vi "Enque(waveforms).vi"(7 "at front (F)":bool, 8 "error in":errorcluster, 9 "Message Payload waveforms":waveform(dbl)[](array[waveform]), 10 "Message Command":string, 11 "Message que":T1) -> (0 "error out":errorcluster, 3 "Message que out":T1)   [LabVIEW 2017]
doc: "Transmit a message with a waveform array payload.\nFor a regular message, enqueue the message. For a priority message, enqueue it at the front of the queue.\n\nBolder Software LLC"
uses:
  MessageQue/MessageQue.ctl
  MessageQue/MessageCluster.ctl
  MessageQue/MessageQue.lvlib
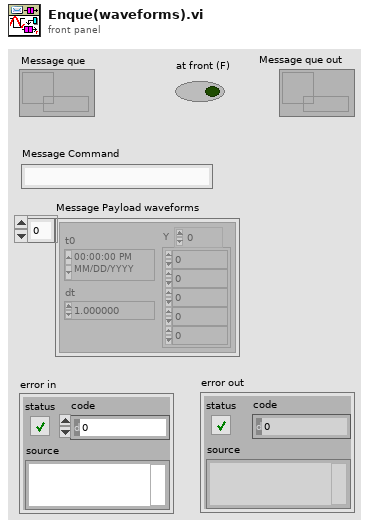
[diagram p1: front panel]
types:
  T1 = typedef "MessageQue.lvlib/MessageQue.ctl" = refnum<queue>
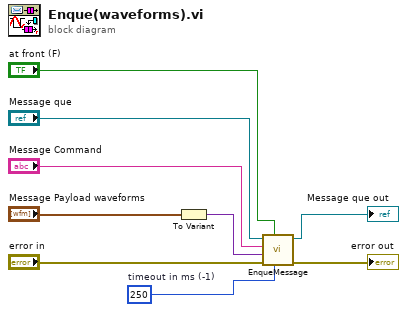
[diagram p0: block diagram]
diagram:
  w9 = 250  # timeout in ms (-1)
  n1 = To Variant(anything="Message Payload waveforms") -> (Variant=w3:variant)
  n2 = call "EnqueMessage.vi"("timeout in ms (-1)"=w9, "Priority Message? (F)"="at front (F)", "error in"="error in", "Message Payload"=w3, "Message Command"="Message Command", "Message que"="Message que") -> ("error out"=→"error out":errorcluster, "Message que out"=→"Message que out":T1)  [unwired: 4 in]
